vi "Tree_Add_Child_to_Bottom.vi"(8 "error in (no error)":errorcluster, 9 "Child String (to add)":string, 10 "Parent Tag":string, 11 "Tree Refnum IN":refnum<vi>) -> (0 "error out":errorcluster, 2 "Newly added Child Tag":string, 3 "Tree Refnum OUT":refnum<vi>)   [LabVIEW 2012]
doc: "SciScan 1.2 160622"
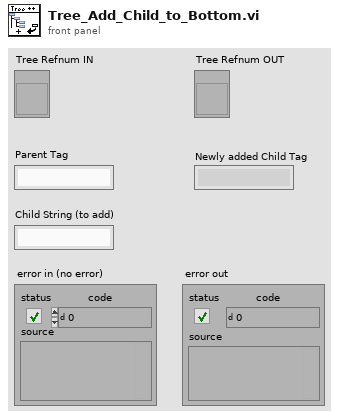
[diagram p1: front panel]
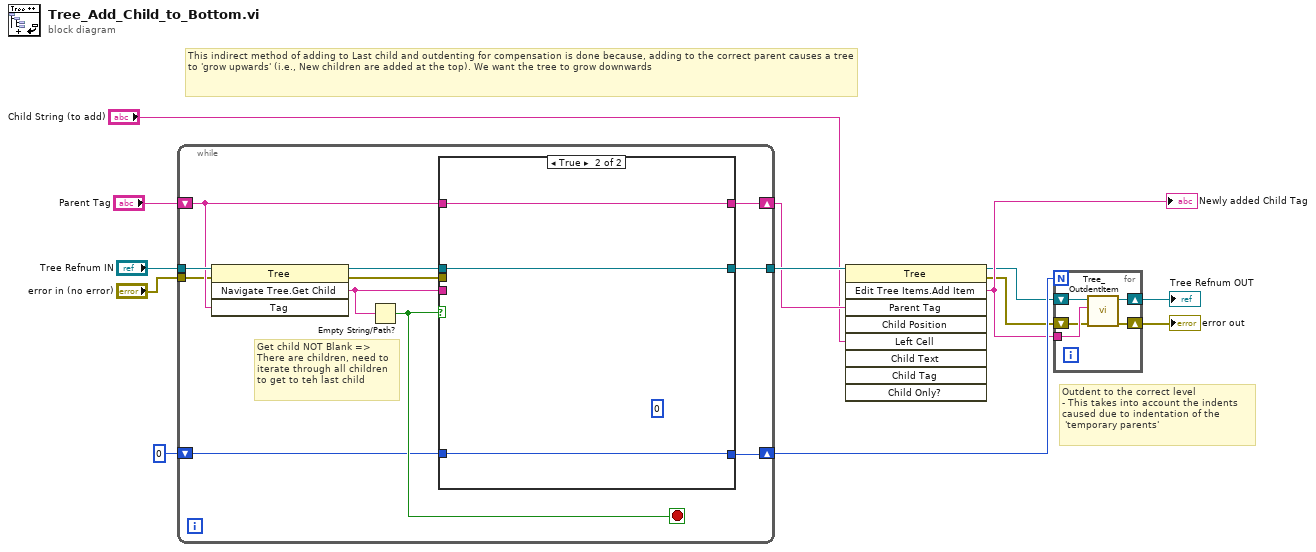
[diagram p0: block diagram]
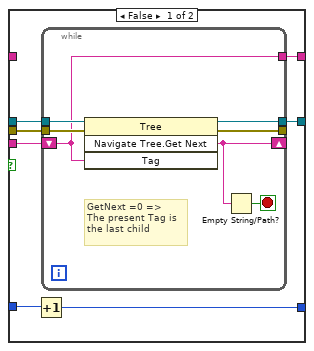
[diagram p2: hidden frame]
diagram:
  # "This indirect method of adding to Last child and outdenting for compensation is done because, adding to the correct parent causes a tree to 'grow upwards' (i.e., New children are added at the top). We want the tree to grow downwards"
  # "Outdent to the correct level\n- This takes into account the indents\ncaused due to indentation of the\n 'temporary parents'"
  n1 = while {
    shift-right: [w20] -> w4
    shift-left: "Parent Tag" -> [w15]
    shift-right: [w18] -> w11
    shift-left: 0 -> [w19]
    tunnel: "Tree Refnum IN" -> [w17]
    tunnel: [w16] -> w7
    tunnel: "error in (no error)" -> [w14]
    stop <- w21 stop-if-true
    # "Get child NOT Blank =>\nThere are children, need to\niterate through all children\nto get to teh last child"
    n2 = invoke class="Tree" method="Navigate Tree.Get Child"(reference=w17, error in=w14, "Tag"=w15) -> (reference out=w23:refnum<vi>, error out=w24:errorcluster, "Navigate Tree:Get Child"=w22:string)  [unwired: 1 in, 1 out]
    n3 = Empty String/Path?(string/path=w22) -> (empty?=w21:bool)
    n4 = case shown="True" w21 {
      tunnel: w24 -> [w31 _]
      tunnel: w23 -> [w30 w41]
      tunnel: w22 -> [w29 _]
      tunnel: [w28 w39] -> w20
      tunnel: w19 -> [w27 w40]
      tunnel: [w26 w40] -> w18
      tunnel: [w25 w41] -> w16
      tunnel: w15 -> [_ w39]
      frame False {
        n5 = Increment(x=w27) -> (x+1=w26:i32)
        n6 = while {
          tunnel: w30 -> [w38]
          shift-right: [w34] -> _
          shift-left: w29 -> [w32]
          tunnel: [w32] -> w28
          tunnel: [w35] -> w25
          tunnel: [w36] -> _
          tunnel: w31 -> [w37]
          stop <- w33 stop-if-true
          # "GetNext =0 =>\nThe present Tag is \nthe last child"
          n7 = invoke class="Tree" method="Navigate Tree.Get Next"(reference=w38, error in=w37, "Tag"=w32) -> (reference out=w35:refnum<vi>, error out=w36:errorcluster, "Navigate Tree:Get Next Item"=w34:string)  [unwired: 1 in, 1 out]
          n8 = Empty String/Path?(string/path=w34) -> (empty?=w33:bool)
        }
      }
      frame True {
        (unwired) 0
      }
    }
  }
  n9 = invoke class="Tree" method="Edit Tree Items.Add Item"(reference=w7, "Parent Tag"=w4, "Left Cell"="Child String (to add)") -> (reference out=w6:refnum<vi>, error out=w5:errorcluster, "Edit Tree Items:Add Item"=w9:string)  [unwired: 6 in, 6 out]
  "Newly added Child Tag" <- w9
  n10 = for {
    N: w11 -> [_]
    tunnel: w9 -> [w46]
    shift-right: [w45] -> w3
    shift-left: w5 -> [w43]
    shift-right: [w44] -> w10
    shift-left: w6 -> [w42]
    n11 = call "Tree_OutdentItem.vi"("Error In"=w43, "TagToOutdent"=w46, "Tree Refnum"=w42) -> ("Error Out"=w45:errorcluster, "Tree Refnum OUT"=w44:refnum<vi>)  [unwired: 7 in]
  }
  "Tree Refnum OUT" <- w10
  "error out" <- w3
